vi "Crée Texte.vi"(3 "Niveaux":dbl, 4 "Temperature":dbl) -> (0 "Texte":string)   [LabVIEW 2022 SP3]
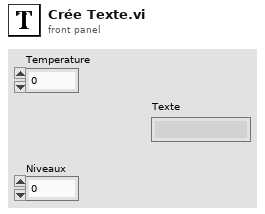
[diagram p1: front panel]
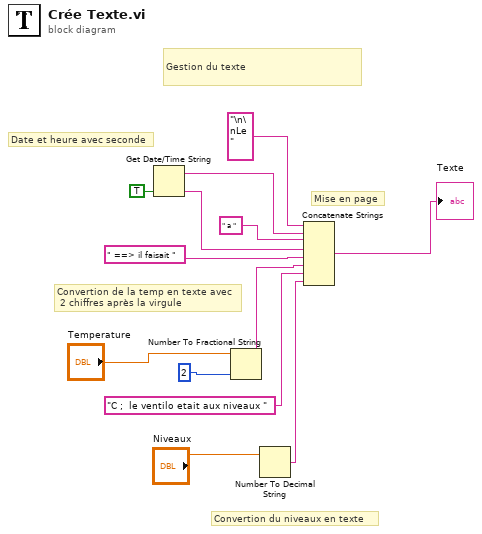
[diagram p0: block diagram]
diagram:
  # "Convertion du niveaux en texte"
  # "Convertion de la temp en texte avec\n 2 chiffres après la virgule"
  # "Date et heure avec seconde"
  # "Mise en page"
  # "Gestion du texte"
  n1 = Get Date/Time String(want seconds? (F)=TRUE) -> (date string=w12:string, time string=w5:string)  [unwired: 2 in]
  n2 = Number To Fractional String(number="Temperature", precision (6)=i16 2) -> (F-format string=w9:string)  [unwired: 2 in]
  n3 = Number To Decimal String(number="Niveaux") -> (decimal integer string=w2:string)  [unwired: 1 in]
  n4 = Concatenate Strings("\n\nLe  " ("string"), w12, " a " ("string"), w5, " ==> il faisait " ("string"), w9, "C ;  le ventilo etait aux niveaux " ("string"), w2) -> (→"Texte":string)
